vi "ILRstripChart.vi"() -> ()   [LabVIEW 2015]
panel:
  in  "Stop Button":bool
  in  "Port Name":string
  out "Waveform Chart":dbl(graph)
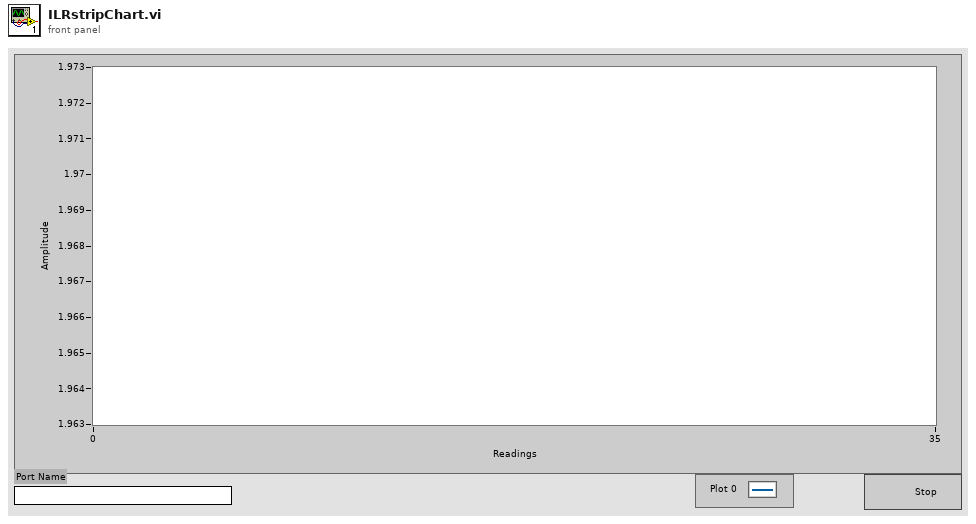
[diagram p1: front panel]
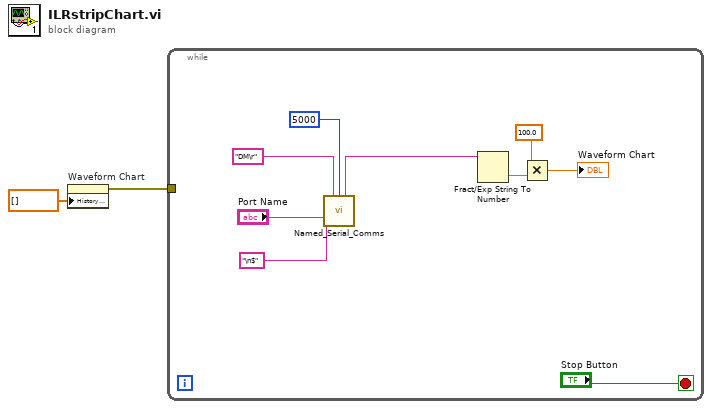
[diagram p0: block diagram]
diagram:
  n1 = property on="Waveform Chart" class="WFChart (strict)"("History Data"=dbl[] []) -> (error out=w1:errorcluster)  [unwired: 2 in, 1 out]
  n2 = while {
    tunnel: w1 -> [_]
    stop <- "Stop Button" stop-if-true
    n3 = call "Named_Serial_Comms.vi"("Write String"="DM\r", "Timeout/ms"=u32 5000, "Port Name"="Port Name", "Term Grep"="\n$") -> ("Read"=w8:string)  [unwired: 8 in, 3 out]
    n4 = Fract/Exp String To Number(string=w8) -> (number=w7:dbl)  [unwired: 3 in, 1 out]
    n5 = Multiply(x=100.0, y=w7) -> (x*y=→"Waveform Chart":dbl)
  }
